vi "继电器控制工况.vi"(0 "tdk":refnum<visa-resource-name>, 1 "6332b":refnum<visa-resource-name>, 2 "Bool引用句柄":refnum<vi>, 5 "error out":errorcluster, 6 "工况1":dbl[][](array[numeric]), 7 "工况2":dbl[][](array[numeric]), 8 "电源台数":dbl=3.0, 10 "大循环次数":i32, 15 "工况1循环次数":i32, 18 "工况2循环次数":i32) -> (3 "完成工况1循环":i32, 11 "已成大循环数":i32, 14 "VISA resource name out":refnum<visa-resource-name>, 17 "完成工况2循环":i32, 19 "错误输出":errorcluster)   [LabVIEW 2021]
uses:
  <instrlib>/TDK-Lambda G Series/TDK-Lambda G Series.lvlib
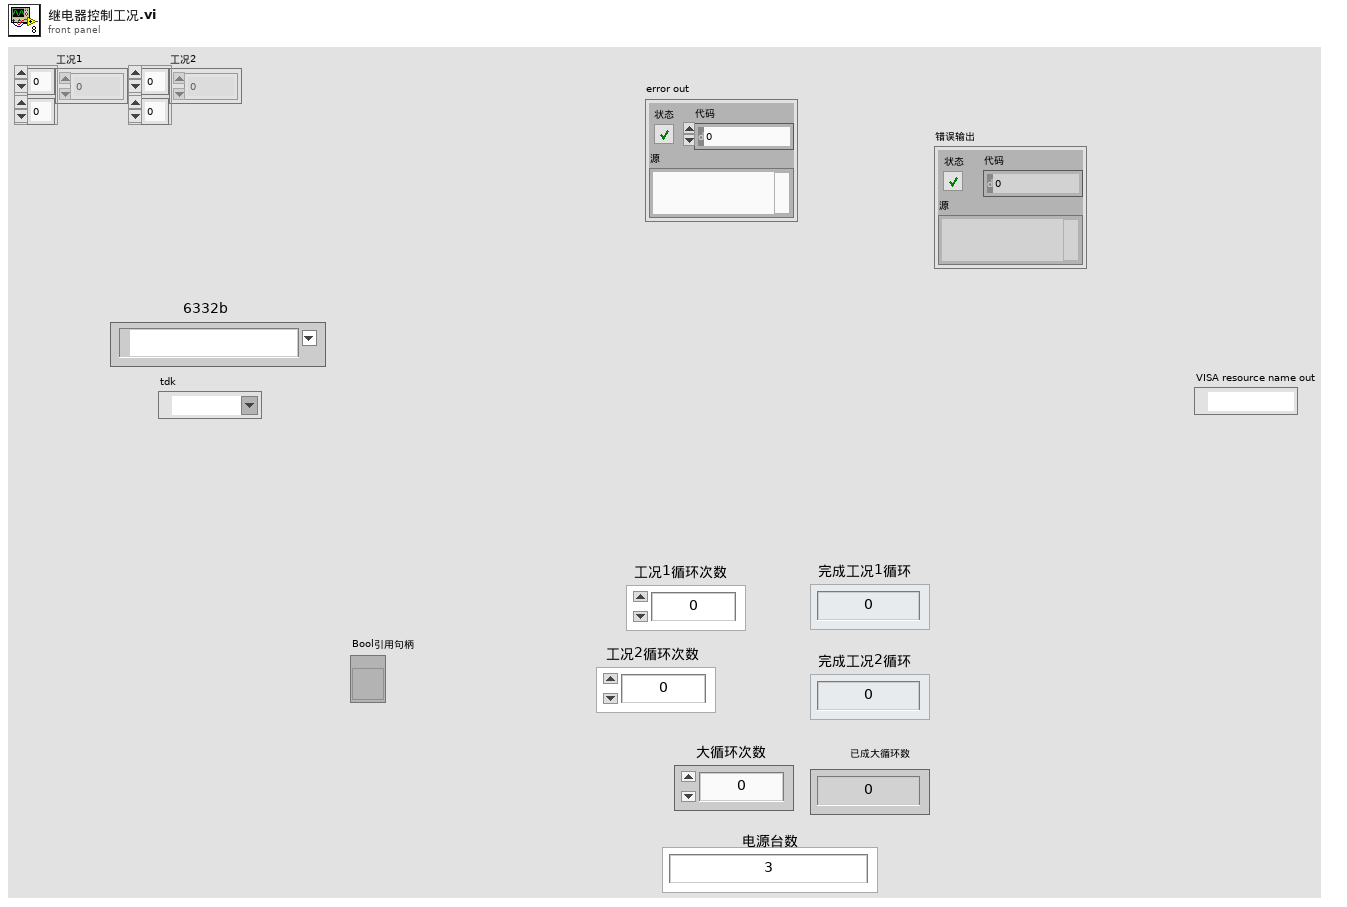
[diagram p1: front panel]
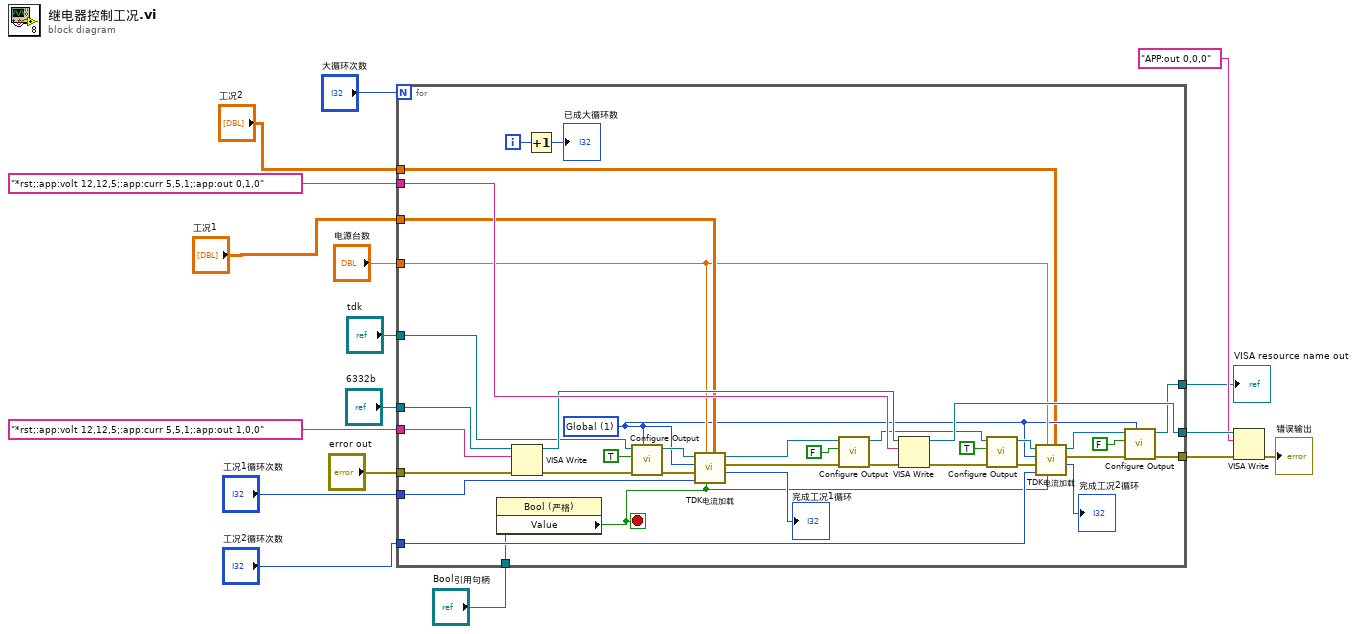
[diagram p0: block diagram]
diagram:
  n1 = for {
    N: "大循环次数" -> [_]
    tunnel: "*rst;:app:volt 12,12,5;:app:curr 5,5,1;:app:out 1,0,0" -> [w54]
    tunnel: "6332b" -> [w53]
    tunnel: "*rst;:app:volt 12,12,5;:app:curr 5,5,1;:app:out 0,1,0" -> [w52]
    tunnel: [w50] -> w17
    tunnel: "tdk" -> [w38]
    tunnel: "工况1" -> [w49]
    tunnel: "error out" -> [w48]
    tunnel: [w32] -> w9
    tunnel: "工况1循环次数" -> [w45]
    tunnel: "工况2循环次数" -> [w44]
    tunnel: [w30] -> w10
    tunnel: "电源台数" -> [w43]
    tunnel: "工况2" -> [w20]
    tunnel: "Bool引用句柄" -> [w19]
    i -> [w22]
    stop <- w18 stop-if-true
    w23 = u16 1 items=["Single", "Global"] ("Globalize (0: Single)")
    n2 = property class="Bool (严格)"(reference=w19) -> ("Value"=w18:bool)  [unwired: 1 in, 2 out]
    n3 = VISA Write(VISA resource name=w53, write buffer=w54, error in (no error)=w48) -> (VISA resource name out=w51:refnum<visa-resource-name>, error out=w42:errorcluster)  [unwired: 1 out]
    n4 = Increment(x=w22) -> (x+1=→"已成大循环数":i32)
    n5 = call <instrlib>:"Configure Output.vi"("Globalize (0: Single)"=w23, "error in (no error)"=w42, "Enable Output (False)"=TRUE, "VISA resource name"=w38) -> ("error out"=w41:errorcluster, "VISA resource name out"=w31:refnum<visa-resource-name>)  [unwired: 6 in]
    n6 = call "TDK电流加载.vi"("all rows"=w49, "停止"=w18, "电源台数"=w43, "循环次数"=w45, "error out"=w41, "Globalize (0: Single)"=w23, "VISA resource name out"=w31) -> ("已完成循环次数"=→"完成工况1循环":i32, "error out 2"=w27:errorcluster, "VISA resource name out 2"=w26:refnum<visa-resource-name>)  [unwired: 2 in]
    n7 = call <instrlib>:"Configure Output.vi"("error in (no error)"=w27, "Enable Output (False)"=FALSE, "VISA resource name"=w26) -> ("error out"=w39:errorcluster, "VISA resource name out"=w29:refnum<visa-resource-name>)  [unwired: 7 in]
    n8 = VISA Write(VISA resource name=w51, write buffer=w52, error in (no error)=w39) -> (VISA resource name out=w50:refnum<visa-resource-name>, error out=w36:errorcluster)  [unwired: 1 out]
    n9 = call <instrlib>:"Configure Output.vi"("error in (no error)"=w36, "Enable Output (False)"=TRUE, "VISA resource name"=w29) -> ("error out"=w35:errorcluster, "VISA resource name out"=w28:refnum<visa-resource-name>)  [unwired: 7 in]
    n10 = call "TDK电流加载.vi"("all rows"=w20, "停止"=w18, "电源台数"=w43, "循环次数"=w44, "error out"=w35, "Globalize (0: Single)"=w23, "VISA resource name out"=w28) -> ("已完成循环次数"=→"完成工况2循环":i32, "error out 2"=w25:errorcluster, "VISA resource name out 2"=w24:refnum<visa-resource-name>)  [unwired: 2 in]
    n11 = call <instrlib>:"Configure Output.vi"("Globalize (0: Single)"=w23, "error in (no error)"=w25, "Enable Output (False)"=FALSE, "VISA resource name"=w24) -> ("error out"=w32:errorcluster, "VISA resource name out"=w30:refnum<visa-resource-name>)  [unwired: 6 in]
  }
  "VISA resource name out" <- w10
  n12 = VISA Write(VISA resource name=w17, write buffer="APP:out 0,0,0" ("写入缓冲区"), error in (no error)=w9) -> (error out=→"错误输出":errorcluster)  [unwired: 2 out]
